vi "Reset.vi"(8 "error in (no error)":errorcluster, 10 "Message in":refnum<class "ResetMessage.lvclass">, 11 "DAQOrcaFlash in":refnum<class "DAQOrcaFlash.lvclass">) -> (0 "error out":errorcluster, 3 "DAQOrcaFlash out":refnum<class "DAQOrcaFlash.lvclass">)   [LabVIEW 2012, in "DAQOrcaFlash.lvclass"]
doc: "The reset method processes the command 'reset'. \n\nResets the internal state of the component (without performing a full initialisation). This could be resetting hardware, or private data to default values."
uses:
  DAQOrcaFlash.lvclass
  <vilib>/Distrio/Murmex/ResetMessage/ResetMessage.lvclass
  <vilib>/Distrio/Murmex/InitialiseMessage/InitialiseMessage.lvclass
  <vilib>/Utility/sysdir.llb/System Directory Type.ctl
  <vilib>/Distrio/Murmex/StopMessage/StopMessage.lvclass
  <vilib>/Distrio/Murmex/GenericMessage/GenericMessage.lvclass
  <vilib>/Distrio/Murmex/Murmex/Murmex.lvclass
  DAQOrcaFlash.lvclass/DAQOrcaFlash.ctl
  <vilib>/Utility/file.llb/Write To Spreadsheet File (DBL).vi
  <vilib>/Distrio/Murmex/Message/Add or replace parameter.vi
panel:
  # "This method is called when the RESET\ntrigger is sent. \n\nOverride this method when your component needs to\nrespond to this trigger. \n\nCall parent for proper implementation"
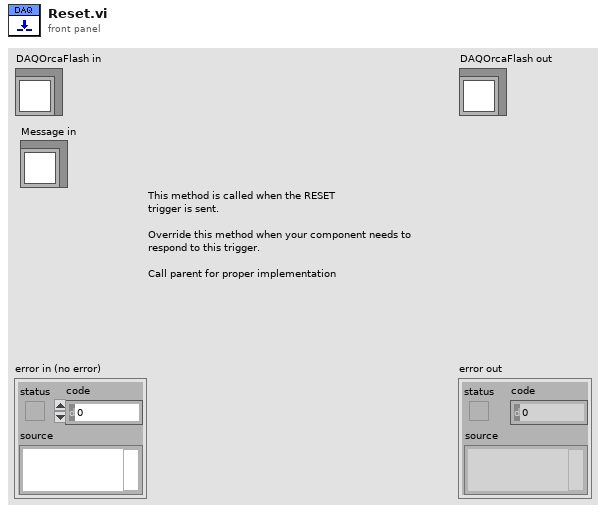
[diagram p1: front panel]
types:
  T1 = typedef "System Directory Type.ctl" = i32
  T2 = typedef "IMAQ Image.ctl" = refnum<image>
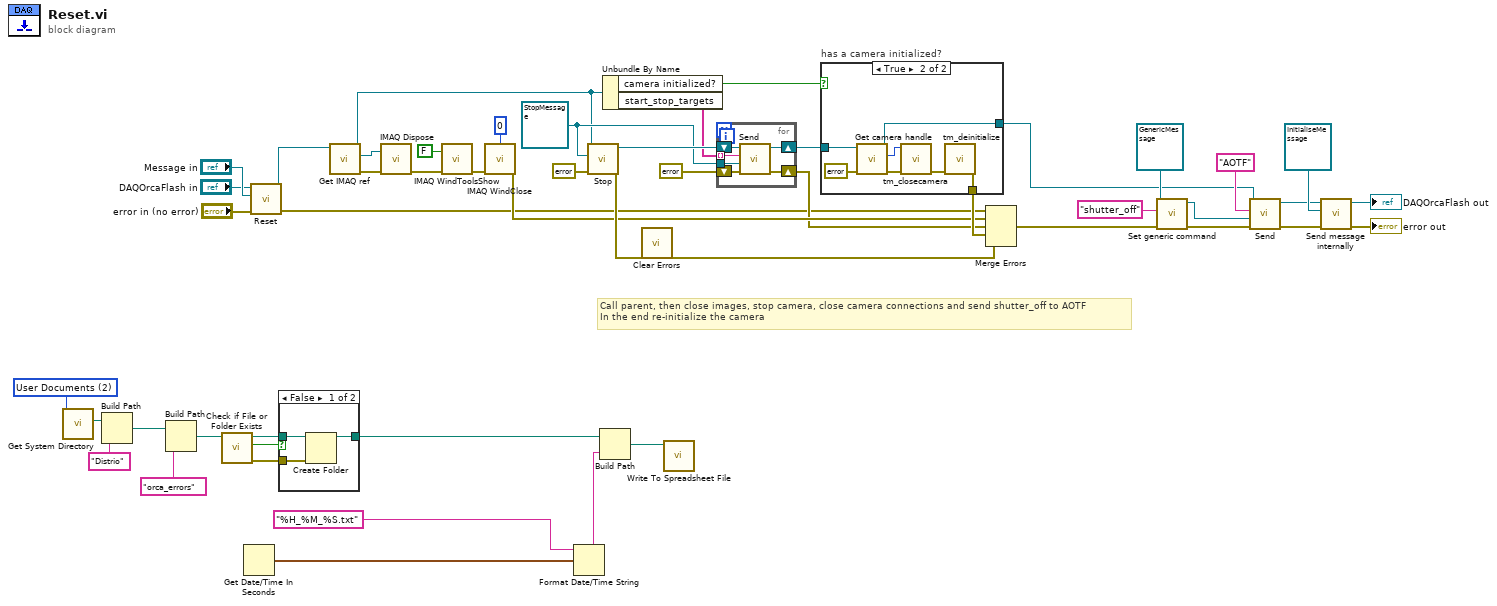
[diagram p0: block diagram]
diagram:
  w14 = refnum<class "StopMessage.lvclass"> refnum ("Message in")
  w41 = T1 2 items=["User Home"=0, "User Desktop"=1, "User Documents"=2, "User Application Data"=3, "User Preferences"=4, "User Temporary"=5, "Public Documents"=6, "Public Application Data"=7, "Public Preferences"=8, "Public Cache"=13, "System Core Libraries"=9, "System Installed Libraries"=10, "Application Files"=11, "Boot Volume Root"=12] ("system directory type")
  # "Call parent, then close images, stop camera, close camera connections and send shutter_off to AOTF\nIn the end re-initialize the camera"
  n1 = call <vilib>:"Get System Directory.vi"("system directory type"=w41) -> ("system directory"=w40:path)  [unwired: 10 in]
  n2 = Build Path(base path=w40, name or relative path="Distrio") -> (appended path=w38:path)
  n3 = Build Path(base path=w38, name or relative path="orca_errors") -> (appended path=w34:path)
  n4 = call <vilib>:"Check if File or Folder Exists.vi"("path"=w34) -> ("error out"=w32:errorcluster, "file or folder exists?"=w31:bool, "dup path"=w35:path)  [unwired: 8 in]
  n5 = Get Date/Time In Seconds() -> (seconds since 1Jan1904=w44:timestamp)
  n6 = call-parent "Reset.vi"("error in (no error)"="error in (no error)", "Message in"="Message in", "Murmex in"="DAQOrcaFlash in") -> ("error out"=w11:errorcluster, "Murmex out"=w10:refnum<class "DAQOrcaFlash.lvclass">)  [unwired: 7 in]
  n7 = case shown="False" w31 {
    tunnel: w35 -> [w53 w54]
    tunnel: [w52 w54] -> w33
    tunnel: w32 -> [w51 _]
    frame False {
      n8 = Create Folder(path (use dialog)=w53, error in=w51) -> (created path=w52:path)  [unwired: 1 in, 2 out]
    }
    frame True {
    }
  }
  n9 = call "Get IMAQ ref.vi"("DAQMH121119OrcaFlash in"=w10) -> ("error out"=w24:errorcluster, "IMAQ reference"=w25:T2, "DAQMH121119OrcaFlash out"=w13:refnum<class "DAQOrcaFlash.lvclass">)  [unwired: 8 in]
  n10 = call "IMAQ Dispose"("Image"=w25, "error in (no error)"=w24) -> ("error out"=w23:errorcluster)  [unwired: 4 in]
  n11 = call "IMAQ WindToolsShow"("Hide/Show (Show)"=FALSE, "error in (no error)"=w23) -> ("error out"=w22:errorcluster)  [unwired: 3 in, 1 out]
  n12 = call "IMAQ WindClose"("Window Number (0...15)"=0, "error in (no error)"=w22) -> ("error out"=w20:errorcluster)  [unwired: 4 in]
  n13 = Format Date/Time String(time format string (%c)="%H_%M_%S.txt", seconds (now)=w44) -> (date/time string=w37:string)  [unwired: 1 in]
  n14 = call-dynamic "Stop.vi"("error in (no error)"=errorcluster {"status"=FALSE, "code"=0, "source"=""}, "Message in"=w14, "DAQMH121119OrcaFlash in"=w13) -> ("error out"=w29:errorcluster, "DAQMH121119OrcaFlash out"=w19:refnum<class "DAQOrcaFlash.lvclass">)  [unwired: 7 in]
  n15 = Build Path(base path=w33, name or relative path=w37) -> (appended path=w36:path)
  n16 = Unbundle By Name(w13) -> ("camera initialized?"=w12:bool, "start_stop_targets"=w16:string[])
  n17 = call <vilib>:"Clear Errors.vi"("error in (no error)"=w29) -> ("error out"=w27:errorcluster)  [unwired: 6 in]
  n18 = call-poly <vilib>:"Write To Spreadsheet File.vi"("file path (dialog if empty)"=w36) -> ()  [unwired: 7 in, 1 out]
  n19 = for {
    tunnel: w16 -> [w57] mode=indexing
    shift-right: [w59] -> w18
    shift-left: w19 -> [w60]
    shift-right: [w56] -> w15
    shift-left: errorcluster {"status"=FALSE, "code"=0, "source"=""} ("error in (no error)") -> [w58]
    tunnel: w14 -> [w55]
    n20 = call <vilib>:"Send.vi"("error in (no error)"=w58, "Message"=w55, "recipient"=w57, "Murmex in"=w60) -> ("error out"=w56:errorcluster, "Murmex out"=w59:refnum<class "DAQOrcaFlash.lvclass">)  [unwired: 6 in]
  }
  n21 = case "has a camera initialized?" shown="True" w12 {
    tunnel: [w61 w68] -> w1
    tunnel: [_ w63] -> w28
    tunnel: w18 -> [w61 w62]
    frame False {
    }
    frame True {
      n22 = call "Get camera handle.vi"("error in (no error)"=errorcluster {"status"=FALSE, "code"=0, "source"=""}, "DAQMH121119OrcaFlash in"=w62) -> ("error out"=w65:errorcluster, "cam handle"=w66:u32, "DAQMH121119OrcaFlash out"=w68:refnum<class "DAQOrcaFlash.lvclass">)  [unwired: 7 in]
      n23 = call <userlib>:"tm_closecamera.vi"("error in (no error)"=w65, "Handle in"=w66) -> ("error out"=w67:errorcluster)  [unwired: 9 in]
      n24 = call <userlib>:"tm_deinitialize.vi"("error in (no error)"=w67) -> ("error out"=w63:errorcluster)  [unwired: 10 in]
    }
  }
  n25 = Merge Errors(w11, w20, w15, w28, w27) -> (w4:errorcluster)
  n26 = call <vilib>:"Set generic command.vi"("error in (no error)"=w4, "generic command"="shutter_off", "GenericMessage in"=refnum<class "GenericMessage.lvclass"> refnum ("Murmex.lvlib:GenericMessage")) -> ("error out"=w8:errorcluster, "GenericMessage out"=w7:refnum<class "GenericMessage.lvclass">)  [unwired: 7 in]
  n27 = call <vilib>:"Send.vi"("error in (no error)"=w8, "Message"=w7, "recipient"="AOTF", "Murmex in"=w1) -> ("error out"=w3:errorcluster, "Murmex out"=w2:refnum<class "DAQOrcaFlash.lvclass">)  [unwired: 6 in]
  n28 = call <vilib>:"Send message internally.vi"("error in (no error)"=w3, "Message"=refnum<class "InitialiseMessage.lvclass"> refnum ("Message in"), "Murmex in"=w2) -> ("error out"=→"error out":errorcluster, "Murmex out"=→"DAQOrcaFlash out":refnum<class "DAQOrcaFlash.lvclass">)  [unwired: 7 in]
